vi "Load Modules.vi"(8 "error in (no error)":errorcluster, 11 "Application Controller in":refnum<class "Application Controller.lvclass">) -> (0 "error out":errorcluster, 3 "Application Controller out":refnum<class "Application Controller.lvclass">)   [LabVIEW 2019, in "Application Controller.lvclass"]
uses:
  Application Controller.lvclass
  C:/GitHub/LabActor/Template Module/Template Module.lvclass
  Menu Control.ctl
  Application Controller.lvclass/Application Controller.ctl
  Monitor Controller/Monitor Controller.lvclass
  Recorders/PID Controller/PID Controller.lvclass
  Recorders/VI Server/VI Server Recorder.lvclass
  Comms/TCP Communications/TCP Communications.lvclass
  Template Module/Template Module.lvclass/Template Module.ctl
  Template Module/Read Name.vi
  Read Startup Configuration.vi
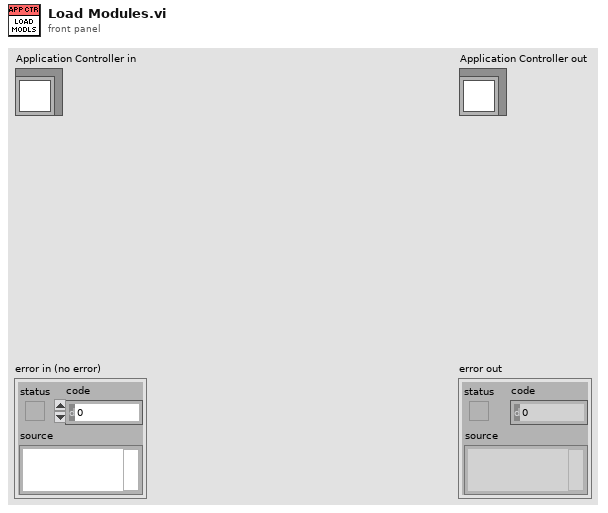
[diagram p1: front panel]
types:
  T1 = typedef "Menu Control.ctl" = enum16{"NONE", "Monitor", "Post-process", "Pulse"}
  T2 = typedef "Start-up Configuration.ctl" = cluster{"Load Modules":T3[], "External Modules Loaders":string[], "Root Data Folder":path}
  T3 = typedef "Module Types.ctl" = enum16{"NONE", "NI-DAQmx", "NI-Scope", "Red Pitaya Digitizer", "GaGe", "VISA Device", "Red Pitaya Lockin", "Monitor Controller", "Pulse Controller", "Integrate Pulse", "Lockin Processor", "File converter", "NHMFL Synthesizer", "Micron Hyperion", "Spectrum Recorder", "Resonance Detector", "TCP Communications", "Format Resonances", "Ruby Spectra", "PID Controller", "Quantum Design", "VI Server"}
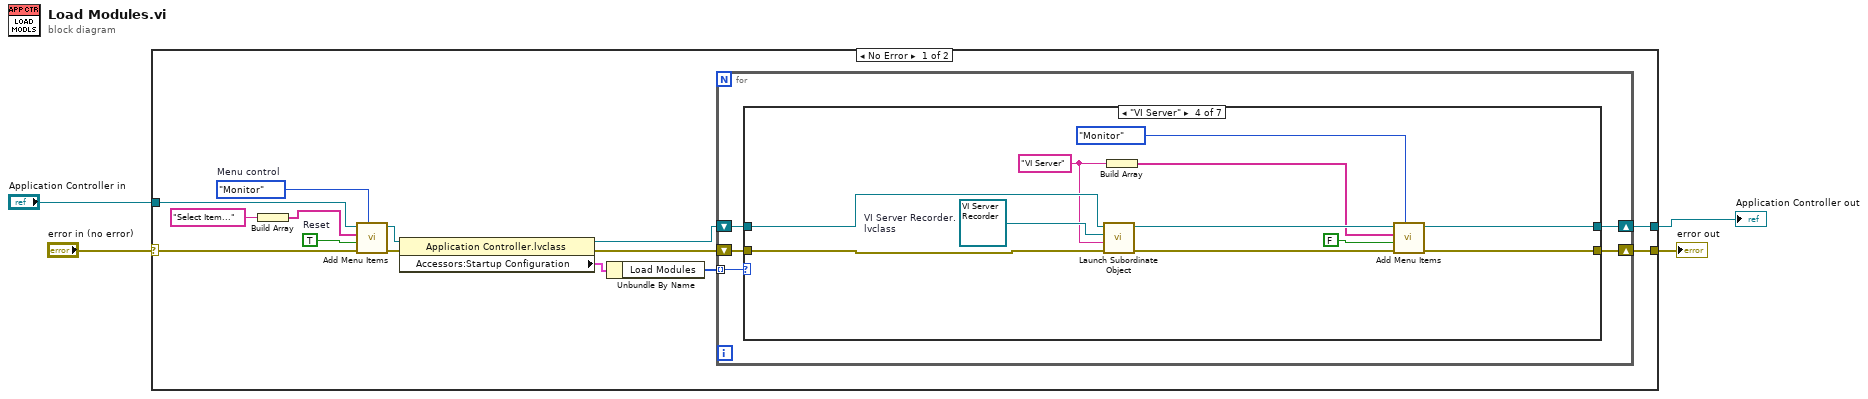
[diagram p0: block diagram]
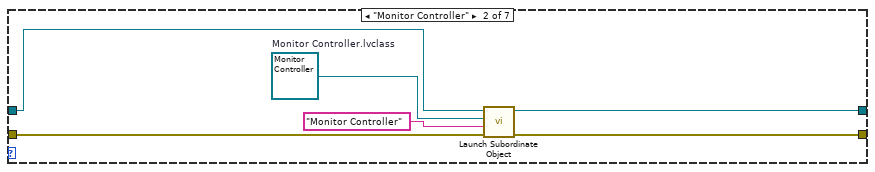
[diagram p3: hidden frame]
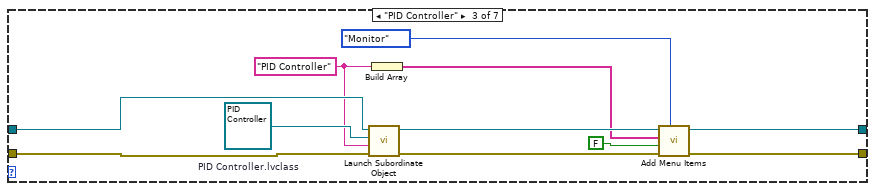
[diagram p4: hidden frame]
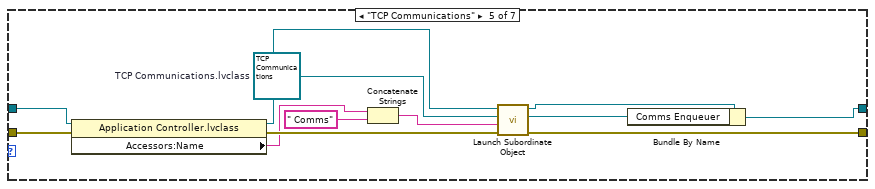
[diagram p5: hidden frame]
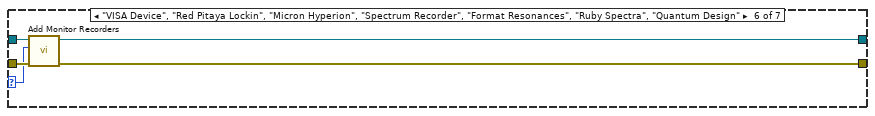
[diagram p6: hidden frame]
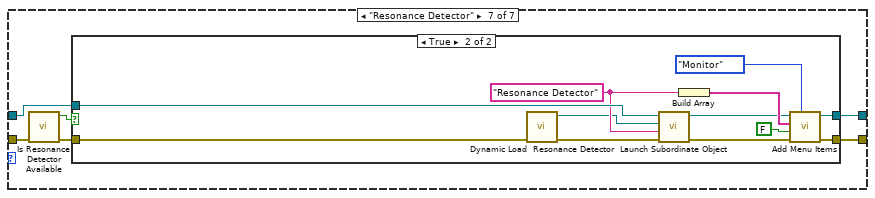
[diagram p7: hidden frame]
diagram:
  n1 = case shown="No Error" "error in (no error)" {
    selector: "error in (no error)" -> [w8 w92]
    tunnel: [w13 w92] -> w3
    tunnel: [w14 w91] -> w1
    tunnel: "Application Controller in" -> [w5 w91]
    frame No Error {
      w7 = Menu_Control."Monitor"  # Menu control
      w11 = TRUE  # Reset
      n2 = Build Array("Select Item..." ("element")) -> (w12:string[])
      n3 = call-dynamic "Add Menu Items.vi"("Menu control"=w7, "error in (no error)"=w8, "Reset"=w11, "Item Names"=w12, "Monitor-Pulse in"=w5) -> ("error out"=w9:errorcluster, "Monitor-Pulse out"=w6:refnum<class "Application Controller.lvclass">)  [unwired: 5 in]
      n4 = property class="Application Controller.lvclass"(reference=w6, error in=w9) -> (reference out=w16:refnum<class "Application Controller.lvclass">, error out=w15:errorcluster, "Accessors:Startup Configuration"=w17:T2)
      n5 = Unbundle By Name(w17) -> ("Load Modules"=w18:T3[])
      n6 = for {
        tunnel: w18 -> [w23] mode=indexing
        shift-right: [w21] -> w13
        shift-left: w15 -> [w22]
        shift-right: [w20] -> w14
        shift-left: w16 -> [w19]
        n7 = case shown="\"VI Server\"" w23 {
          selector: w23 -> [_ _ _ _ _ w66 _]
          tunnel: w22 -> [w24 w29 w41 w52 w64 w70 w72]
          tunnel: [w24 w28 w35 w46 w63 w69 w75] -> w21
          tunnel: w19 -> [w25 w31 w42 w53 w60 w68 w76]
          tunnel: [w25 w30 w36 w47 w55 w67 w74] -> w20
          frame "NONE", Default {
          }
          frame "Monitor Controller" {
            w27 = refnum<class "Monitor Controller.lvclass"> refnum  # Monitor Controller.lvclass
            n8 = call-dynamic "Launch Subordinate Object.vi"("error in (no error)"=w29, "Name"="Monitor Controller", "Subordinate Object"=w27, "Measure Object in"=w31) -> ("error out"=w28:errorcluster, "Measure Object out"=w30:refnum<class "Application Controller.lvclass">)  [unwired: 5 in, 1 out]
          }
          frame "PID Controller" {
            w33 = "PID Controller" ("Name")
            w40 = refnum<class "PID Controller.lvclass"> refnum  # PID Controller.lvclass
            n9 = call-dynamic "Launch Subordinate Object.vi"("error in (no error)"=w41, "Name"=w33, "Subordinate Object"=w40, "Measure Object in"=w42) -> ("error out"=w34:errorcluster, "Measure Object out"=w37:refnum<class "Application Controller.lvclass">)  [unwired: 5 in, 1 out]
            n10 = Build Array(w33) -> (w32:string[])
            n11 = call-dynamic "Add Menu Items.vi"("Menu control"=Menu_Control."Monitor", "error in (no error)"=w34, "Reset"=FALSE, "Item Names"=w32, "Monitor-Pulse in"=w37) -> ("error out"=w35:errorcluster, "Monitor-Pulse out"=w36:refnum<class "Application Controller.lvclass">)  [unwired: 5 in]
          }
          frame "VI Server" {
            w44 = "VI Server" ("Name")
            w51 = refnum<class "VI Server Recorder.lvclass"> refnum  # VI Server Recorder.lvclass
            n12 = call-dynamic "Launch Subordinate Object.vi"("error in (no error)"=w52, "Name"=w44, "Subordinate Object"=w51, "Measure Object in"=w53) -> ("error out"=w45:errorcluster, "Measure Object out"=w48:refnum<class "Application Controller.lvclass">)  [unwired: 5 in, 1 out]
            n13 = Build Array(w44) -> (w43:string[])
            n14 = call-dynamic "Add Menu Items.vi"("Menu control"=Menu_Control."Monitor", "error in (no error)"=w45, "Reset"=FALSE, "Item Names"=w43, "Monitor-Pulse in"=w48) -> ("error out"=w46:errorcluster, "Monitor-Pulse out"=w47:refnum<class "Application Controller.lvclass">)  [unwired: 5 in]
          }
          frame "TCP Communications" {
            w62 = refnum<class "TCP Communications.lvclass"> refnum  # TCP Communications.lvclass
            n15 = property class="Application Controller.lvclass"(reference=w60, error in=w64) -> (reference out=w59:refnum<class "Application Controller.lvclass">, error out=w61:errorcluster, "Accessors:Name"=w58:string)
            n16 = Concatenate Strings(w58, " Comms" ("Name")) -> (w56:string)
            n17 = call-dynamic "Launch Subordinate Object.vi"("error in (no error)"=w61, "Name"=w56, "Subordinate Object"=w62, "Measure Object in"=w59) -> ("error out"=w63:errorcluster, "Nested Actor's Enqueuer"=w54:refnum<class "Message Enqueuer.lvclass">, "Measure Object out"=w65:refnum<class "Application Controller.lvclass">)  [unwired: 5 in]
            n18 = Bundle By Name(cluster=w65, "Comms Enqueuer"=w54) -> (w55:refnum<class "Application Controller.lvclass">)
          }
          frame "VISA Device", "Red Pitaya Lockin", "Micron Hyperion", "Spectrum Recorder", "Format Resonances", "Ruby Spectra", "Quantum Design" {
            n19 = call-dynamic "Add Monitor Recorders.vi"("error in (no error)"=w70, "Module type"=w66, "Monitor-Pulse in"=w68) -> ("error out"=w69:errorcluster, "Monitor-Pulse out"=w67:refnum<class "Application Controller.lvclass">)  [unwired: 6 in, 1 out]
          }
          frame "Resonance Detector" {
            n20 = call "Is Resonance Detector Available.vi"("Error In"=w72) -> ("Error Out"=w71:errorcluster, "Good"=w73:bool)  [unwired: 8 in, 1 out]
            n21 = case shown="True" w73 {
              tunnel: w71 -> [w77 w81]
              tunnel: w76 -> [w78 w90]
              tunnel: [w77 w86] -> w75
              tunnel: [w78 w83] -> w74
              frame False {
              }
              frame True {
                w89 = "Resonance Detector" ("Name")
                n22 = call "Dynamic Load  Resonance Detector.vi"("Error In"=w81) -> ("Error Out"=w80:errorcluster, "Module"=w79:refnum<class "Template Module.lvclass">)  [unwired: 9 in]
                n23 = call-dynamic "Launch Subordinate Object.vi"("error in (no error)"=w80, "Name"=w89, "Subordinate Object"=w79, "Measure Object in"=w90) -> ("error out"=w87:errorcluster, "Measure Object out"=w84:refnum<class "Application Controller.lvclass">)  [unwired: 5 in, 1 out]
                n24 = Build Array(w89) -> (w88:string[])
                n25 = call-dynamic "Add Menu Items.vi"("Menu control"=Menu_Control."Monitor", "error in (no error)"=w87, "Reset"=FALSE, "Item Names"=w88, "Monitor-Pulse in"=w84) -> ("error out"=w86:errorcluster, "Monitor-Pulse out"=w83:refnum<class "Application Controller.lvclass">)  [unwired: 5 in]
              }
            }
          }
        }
      }
    }
    frame Error {
    }
  }
  "error out" <- w3
  "Application Controller out" <- w1
